vi "Time Benchmarking.vi"(10 "Input variable 2":dbl, 11 "Input Variable":dbl) -> (1 "Result":string, 2 "Labview function(ms)":dbl, 3 "Formula Node(ms)":dbl)   [LabVIEW 2014]
doc: "Comparases the execution time for Formula Node and Labview elements for 100,000 iterations and gives th e average time taken.Also displays which ois faster."
panel:
  out "sin(x)":dbl
  out "Sin(x)":dbl
  # "Time Benchamrking"
  # "Runs for 1 Million iterations and compares run time."
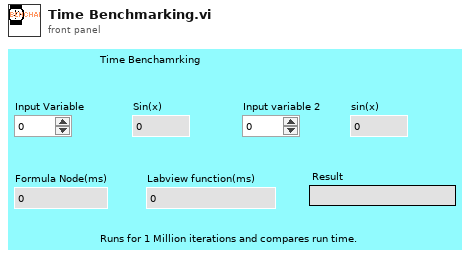
[diagram p1: front panel]
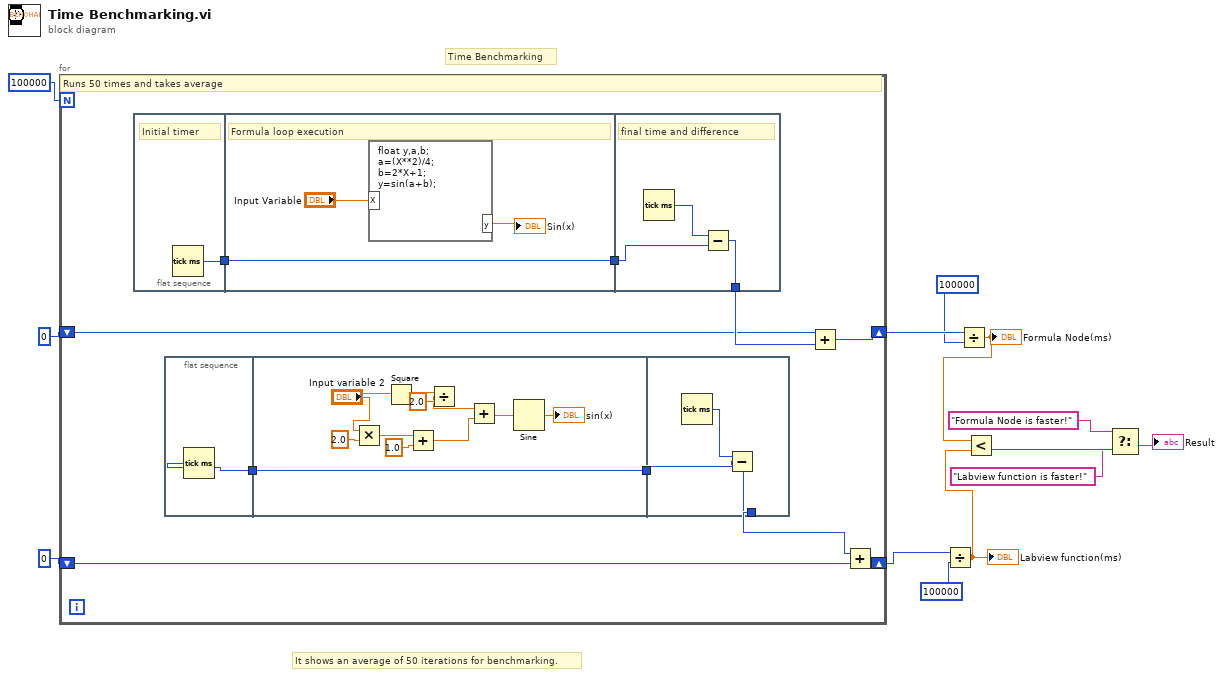
[diagram p0: block diagram]
diagram:
  # "It shows an average of 50 iterations for benchmarking."
  # "Time Benchmarking"
  n1 = for {
    N: 100000 -> [_]
    shift-right: [w20] -> w11
    shift-left: u32 0 -> [w19]
    shift-right: [w15] -> w9
    shift-left: u32 0 -> [w14]
    # "Runs 50 times and takes average"
    n2 = flat-sequence {
      tunnel: [w39] -> w23
      tunnel: [w41] -> w22
      tunnel: w23 -> [w41]
      tunnel: w22 -> [w45]
      tunnel: [w43] -> w21
      frame #0 {
        # "Initial timer"
        n3 = Tick Count (ms)() -> (millisecond timer value=w39:u32)
      }
      frame #1 {
        # "Formula loop execution"
        n4 = formula code="float y,a,b;\na=(X**2)/4;\nb=2*X+1;\ny=sin(a+b);"("X"="Input Variable") -> ("y"=→"Sin(x)":dbl)
      }
      frame #2 {
        # "final time and difference"
        n5 = Tick Count (ms)() -> (millisecond timer value=w44:u32)
        n6 = Subtract(x=w44, y=w45) -> (x-y=w43:u32)
      }
    }
    n7 = flat-sequence {
      tunnel: [w24] -> w17
      tunnel: [w33] -> w18
      tunnel: w17 -> [w33]
      tunnel: w18 -> [w38]
      tunnel: [w36] -> w16
      frame #0 {
        n8 = Tick Count (ms)() -> (millisecond timer value=w24:u32)
      }
      frame #1 {
        n9 = Multiply(x="Input variable 2", y=2.0) -> (x*y=w30:dbl)
        n10 = Square(x="Input variable 2") -> (x^2=w35:dbl)
        n11 = Add(x=w30, y=1.0) -> (x+y=w26:dbl)
        n12 = Divide(x=w35, y=2.0) -> (x/y=w27:dbl)
        n13 = Add(x=w27, y=w26) -> (x+y=w28:dbl)
        n14 = Sine(x=w28) -> (sin(x)=→"sin(x)":dbl)
      }
      frame #2 {
        n15 = Tick Count (ms)() -> (millisecond timer value=w37:u32)
        n16 = Subtract(x=w37, y=w38) -> (x-y=w36:u32)
      }
    }
    n17 = Add(x=w19, y=w21) -> (x+y=w20:u32)
    n18 = Add(x=w16, y=w14) -> (x+y=w15:u32)
  }
  n19 = Divide(x=w9, y=u32 100000) -> (x/y=w5:dbl)
  "Labview function(ms)" <- w5
  n20 = Divide(x=w11, y=u32 100000) -> (x/y=w6:dbl)
  "Formula Node(ms)" <- w6
  n21 = Less?(x=w6, y=w5) -> (x < y?=w4:bool)
  n22 = Select(t="Formula Node is faster!", s=w4, f="Labview function is faster!") -> (s? t:f=→"Result":string)
